vi "quit_reset_VI.vi"(0 "Controls":T1, 3 "error in":errorcluster, 4 "notifier":refnum<notifier>) -> (10 "error out":errorcluster)   [LabVIEW 2016]
uses:
  Type Definitions/control_references.ctl
  Type Definitions/vars_settings.ctl
  Type Definitions/stim_type.ctl
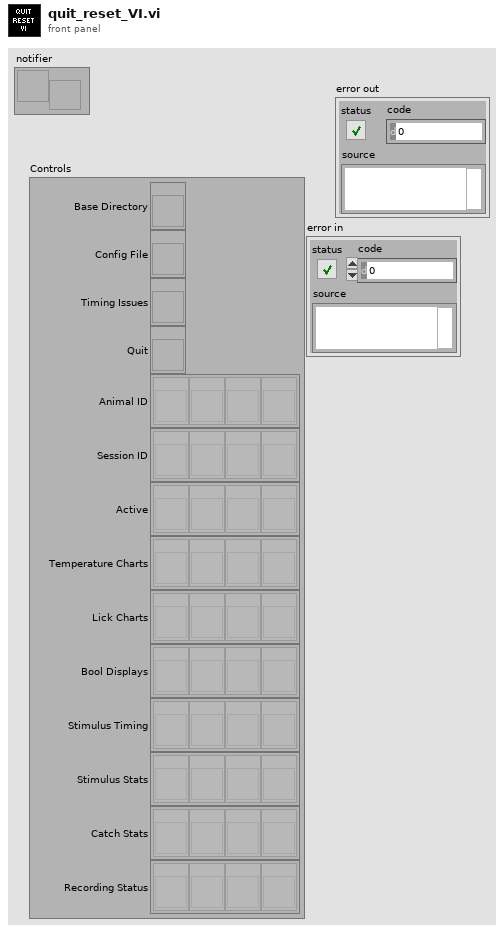
[diagram p1: front panel]
types:
  T1 = typedef "control_references.ctl" = cluster{"Base Directory":refnum<vi>, "Config File":refnum<vi>, "Timing Issues":refnum<vi>, "Quit":refnum<vi>, "Animal ID":refnum<vi>[], "Session ID":refnum<vi>[], "Active":refnum<vi>[], "Temperature Charts":refnum<vi>[], "Lick Charts":refnum<vi>[], "Bool Displays":refnum<vi>[], "Stimulus Timing":refnum<vi>[], "Stimulus Stats":refnum<vi>[], "Catch Stats":refnum<vi>[], "Recording Status":refnum<vi>[]}
  T2 = enum8{"Enabled", "Disabled", "Disabled and Grayed Out"}
  T3 = typedef "vars_settings.ctl" = cluster{"base directory":path, "data directory":path, "active":bool, "running":bool, "pairing":bool, "clean tubes":bool, "animal ID":u16, "session ID":u16, "base temp":dbl, "d wait min":u16, "d wait max":u16, "d timeout":u16, "d reward":u16, "idx stim":u16, "timeout win":u16, "lick win":i32[], "stim type":T4[], "stim dur":u16[], "stim amp":dbl[], "stim freq":u16[], "stim ramp":u16[], "stim catch":u8[], "square dur":u8[], "square delay":u8[], "square freq":u8[], "square dc":u8[], "stim shape":dbl[][], "square shape":bool[][]}
  T4 = typedef "stim_type.ctl" = enum16{"pulse", "vibration", "square", "sine"}
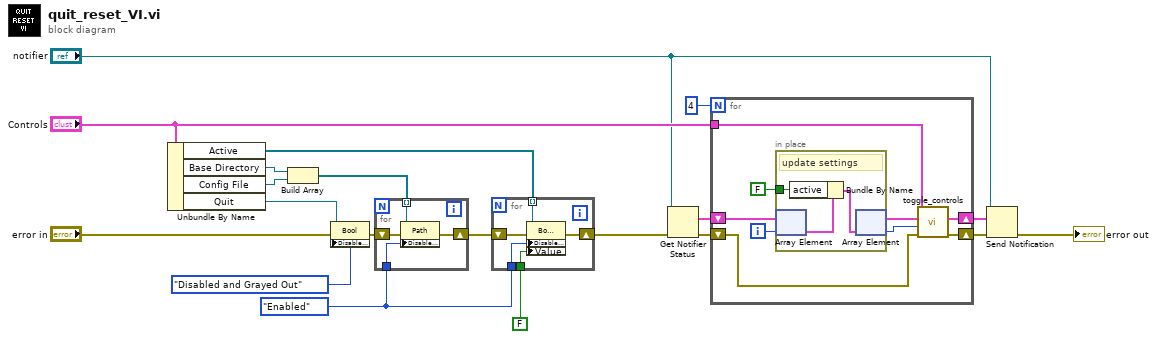
[diagram p0: block diagram]
diagram:
  w5 = T2."Enabled" ("Disabled")
  n1 = Unbundle By Name("Controls") -> ("Active"=w12:refnum<vi>[], "Base Directory"=w17:refnum<vi>, "Config File"=w16:refnum<vi>, "Quit"=w19:refnum<vi>)
  n2 = Build Array(w17, w16) -> (w15:refnum<vi>[])
  n3 = property class="Bool"(reference=w19, error in="error in", "DisabledEnum"=T2."Disabled and Grayed Out" ("Disabled")) -> (error out=w14:errorcluster)  [unwired: 1 out]
  n4 = for {
    tunnel: w15 -> [w23] mode=indexing
    shift-right: [w22] -> w13
    shift-left: w14 -> [w24]
    tunnel: w5 -> [w21]
    n5 = property class="Path"(reference=w23, error in=w24, "DisabledEnum"=w21) -> (error out=w22:errorcluster)  [unwired: 1 out]
  }
  n6 = for {
    shift-right: [w28] -> w6
    shift-left: w13 -> [w27]
    tunnel: w12 -> [w29] mode=indexing
    tunnel: FALSE ("Value") -> [w26]
    tunnel: w5 -> [w25]
    n7 = property class="Bool (strict)"(reference=w29, error in=w27, "DisabledEnum"=w25, "Value"=w26) -> (error out=w28:errorcluster)  [unwired: 1 out]
  }
  n8 = Get Notifier Status(notifier="notifier", error in (no error)=w6) -> (current notification=w10:T3[], error out=w8:errorcluster)  [unwired: 3 out]
  n9 = for "toggle controls" {
    N: 4 -> [_]
    shift-right: [w38] -> w4
    shift-left: w8 -> [w31]
    tunnel: "Controls" -> [w36]
    shift-right: [w37] -> w1
    shift-left: w10 -> [w35]
    i -> [w32]
    n10 = in-place {
      in-place-border: FALSE -> [w40]
      # "update settings"
      n11 = in-place-array #1(w35, w32) -> (w41:T3)
      n12 = Bundle By Name(cluster=w41, "active"=w40) -> (w39:T3)
      n13 = in-place-array #1(w39) -> (w34:T3[], w33:i32)
    }
    n14 = call "toggle_controls.vi"("error in"=w31, "setup ID"=w33, "vars general in"=w34, "control cluster in"=w36) -> ("error out"=w38:errorcluster, "vars general out"=w37:T3[])  [unwired: 4 in, 2 out]
  }
  n15 = Send Notification(notification=w1, notifier="notifier", error in (no error)=w4) -> (error out=→"error out":errorcluster)  [unwired: 1 out]
